vi "Remove Header.vi"(8 "error in (no error)":errorcluster, 10 "Header":string, 11 "Response in":refnum<class "Response.lvclass">) -> (0 "error out":errorcluster, 1 "Value":string, 2 "Removed?":bool, 3 "Response out":refnum<class "Response.lvclass">)   [LabVIEW 2020, in "HTTP Utils.lvlib" / "Response.lvclass"]
uses:
  Response.lvclass
  Response.lvclass/Response.ctl
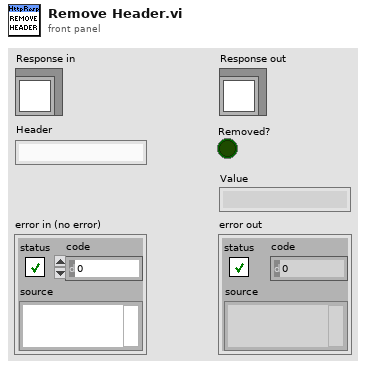
[diagram p1: front panel]
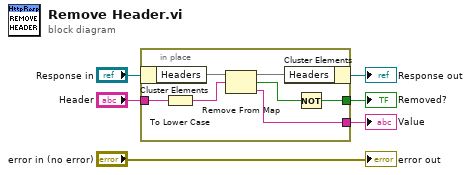
[diagram p0: block diagram]
diagram:
  n1 = in-place {
    in-place-border: "Header" -> [w12]
    in-place-border: [w9] -> w2
    in-place-border: [w8] -> w1
    n2 = in-place-cluster #1("Response in") -> ("Headers"=w13:map{string, string})
    n3 = To Lower Case(string=w12) -> (all lower case string=w7:string)
    n4 = Remove From Map(10:w7, 11:w13) -> (1:w8:string, 2:w10:bool, 3:w11:map{string, string})
    n5 = in-place-cluster #1("Headers"=w11) -> (→"Response out":refnum<class "Response.lvclass">)
    n6 = Not(x=w10) -> (.not. x?=w9:bool)
  }
  "Removed?" <- w2
  "Value" <- w1
  "error out" <- "error in (no error)"
